vi "Diff Remote-Local.vi"(8 "error in (no error)":errorcluster, 11 "Artifactory.VIPM in":refnum<class "Artifactory.VIPM.lvclass">) -> (0 "error out":errorcluster, 1 "has Changes?":bool, 2 "DIff":map{string, string[]}(c390), 3 "Artifactory.VIPM out":refnum<class "Artifactory.VIPM.lvclass">)   [LabVIEW 2021, in "Artifactory.VIPM.lvclass"]
uses:
  Artifactory.VIPM.lvclass
  Artifactory.VIPM.lvclass/Artifactory.VIPM.ctl
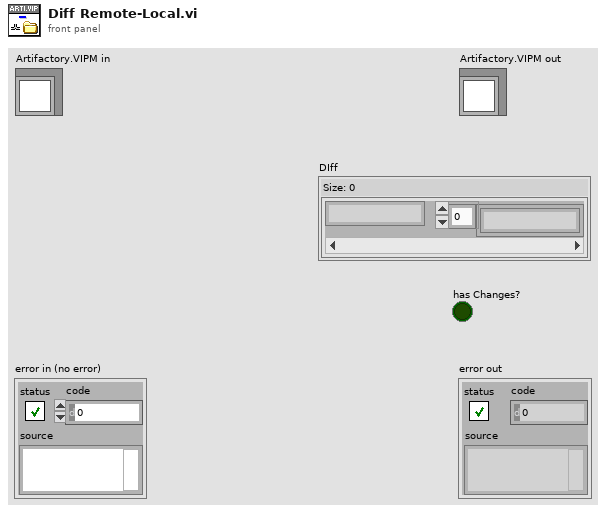
[diagram p1: front panel]
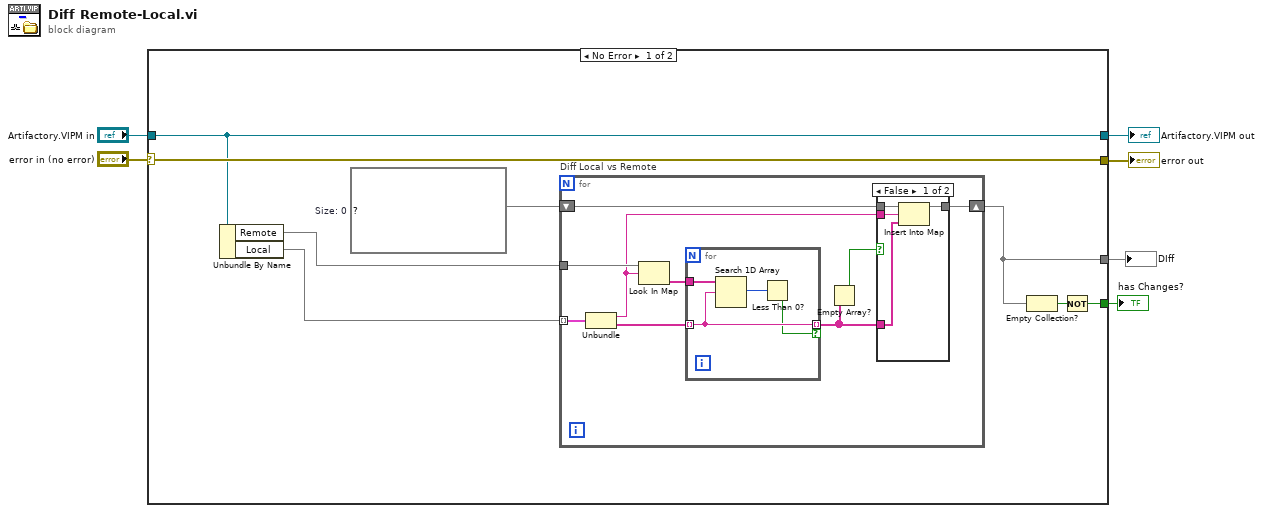
[diagram p0: block diagram]
diagram:
  n1 = case shown="No Error" "error in (no error)" {
    selector: "error in (no error)" -> [w11 w34]
    tunnel: [w11 w34] -> w5
    tunnel: [w10 w33] -> w3
    tunnel: "Artifactory.VIPM in" -> [w10 w33]
    tunnel: [w9 _] -> w2
    tunnel: [w7 _] -> w1
    frame No Error {
      w14 = map{string, string[]} {}  # Size: 0
      n2 = Unbundle By Name(w10) -> ("Remote"=w13:map{string, string[]}, "Local"=w12:map{string, string[]})
      n3 = for "Diff Local vs Remote" {
        tunnel: w13 -> [w23]
        tunnel: w12 -> [w22] mode=indexing
        shift-right: [w18] -> w9
        shift-left: w14 -> [w17]
        n4 = Unbundle(w22) -> ("package_name"=w16:string, "versions"=w21:string[])
        n5 = Look In Map(map=w23, key=w16) -> (value=w20:string[])  [unwired: 1 in, 1 out]
        n6 = for {
          tunnel: w21 -> [w30] mode=indexing
          tunnel: w20 -> [w32]
          tunnel: [w30] -> w15 mode=indexing if=w29
          n7 = Search 1D Array(1D array=w32, element=w30) -> (index of element=w31:i32)  [unwired: 1 in]
          n8 = Less Than 0?(x=w31) -> (x < 0?=w29:bool)
        }
        n9 = Empty Array?(array=w15) -> (empty?=w19:bool)
        n10 = case shown="False" w19 {
          tunnel: [w26 w28] -> w18
          tunnel: w17 -> [w27 w28]
          tunnel: w16 -> [w25 _]
          tunnel: w15 -> [w24 _]
          frame False {
            n11 = Insert Into Map(map in=w27, key=w25, value=w24) -> (map out=w26:map{string, string[]})  [unwired: 2 out]
          }
          frame True {
          }
        }
      }
      n12 = Empty Collection?(1:w9) -> (0:w8:bool)
      n13 = Not(x=w8) -> (.not. x?=w7:bool)
    }
    frame Error {
    }
  }
  "error out" <- w5
  "Artifactory.VIPM out" <- w3
  "DIff" <- w2
  "has Changes?" <- w1
